vi "_Check range DBL.vi"(6 "Error Mode (Errors)":enum16{"Errors Off", "Errors", "Warnings"}(ring)=enum."Errors", 7 "Range Table Identifier":string, 8 "error in (no error)":errorcluster, 10 "DBL Value In":dbl, 11 "VISA resource name":refnum<visa-resource-name>) -> (0 "error out":errorcluster, 2 "DBL Value Out":dbl, 3 "VISA resource name out":refnum<visa-resource-name>)   [LabVIEW 2015, in "Rohde&Schwarz CMXP NR FR2 Measurement.lvlib"]
uses:
  <instrlib>/Rohde&Schwarz CMXP NR FR2 Measurement/Rohde&Schwarz CMXP NR FR2 Measurement.lvlib
  <instrlib>/Rohde&Schwarz CMXP NR FR2 Measurement/Private/rsidr_core.llb/type_Error_Codes.ctl
  <instrlib>/Rohde&Schwarz CMXP NR FR2 Measurement/Public/Utility/rsidr_core_global.vi
  <instrlib>/Rohde&Schwarz CMXP NR FR2 Measurement/Private/rsidr_core.llb/rsidr_core.lvlib
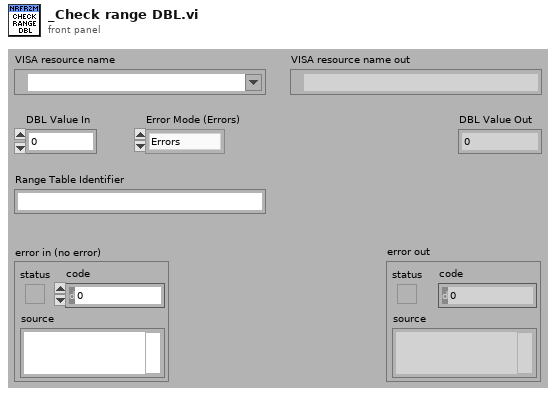
[diagram p1: front panel]
types:
  T1 = typedef "Rohde&Schwarz CMXP NR FR2 Measurement.lvlib/rsidr_core.lvlib/type_Error_Codes.ctl" = enum16{"No_error", "VISA_err_ResourceNotFound", "VISA_err_Timeout", "VISA_warn_MoreDataAvailable", "RS_err_MissingCallback", "RS_err_InvalidAttribute", "RS_err_InvalidValue", "RS_err_UnknownResource", "RS_err_AlreadyInitialized", "RS_err_InstrumentStatus", "RS_err_BadRepCapName", "RS_err_TypesMismatch", "RS_err_ValueNotSupported", "RS_err_InvalidRngTable", "RS_err_IDqueryFail", "RS_err_UnexpResponse", "VISA_warn_ConfigNotLoaded", "RS_err_AttributeNotReadable", "RS_err_AttributeNotWritable", "RS_err_InstrumentType", "RS_err_InstrumentOption", "VISA_err_InvalidSize", "RS_err_ReliabilityIndicator", "VISA_warn_UnknownStatus", "VISA_warn_TermCharRead", "VISA_err_IO_error", "RS_err_FunctionNotSupported", "VISA_warn_QueueEmpty"}
  T2 = cluster{"Name":string, "Type":enum16{"Range", "Coerced", "Discrete"}, "Entries":cluster{"Name":string, "Discrete or Min":dbl, "Max":dbl, "Coerced":dbl, "Command":string}[]}[]
  T3 = cluster{"Name":string, "Discrete or Min":dbl, "Max":dbl, "Coerced":dbl, "Command":string}[]
  T4 = cluster{"Name":string, "Discrete or Min":dbl, "Max":dbl, "Coerced":dbl, "Command":string}
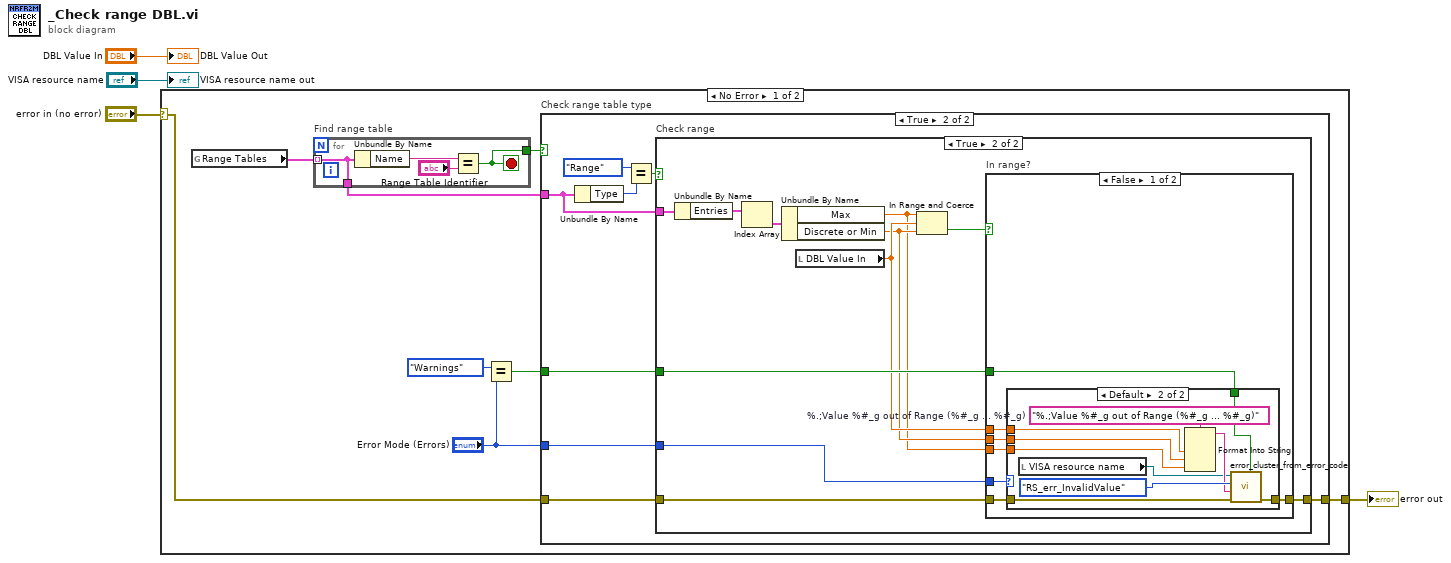
[diagram p0: block diagram]
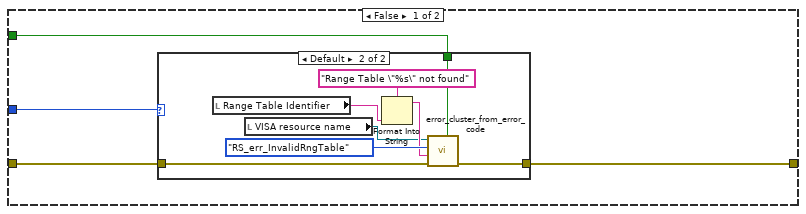
[diagram p2: hidden frame]
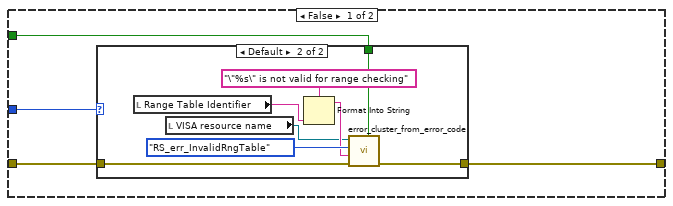
[diagram p4: hidden frame]
diagram:
  n1 = case shown="No Error" "error in (no error)" {
    selector: "error in (no error)" -> [w9 w81]
    tunnel: [w8 w81] -> w2
    frame No Error {
      n2 = global read "rsidr_core_global.vi" "Range Tables"() -> (w12:T2)
      n3 = for "Find range table" {
        tunnel: w12 -> [w78] mode=indexing
        tunnel: [w78] -> w11
        tunnel: [w77] -> w10
        stop <- w77 stop-if-true
        n4 = Unbundle By Name(w78) -> ("Name"=w79:string)
        n5 = Equal?(x=w79, y="Range Table Identifier") -> (x = y?=w77:bool)
      }
      n6 = Equal?(x=enum16{"Errors Off", "Errors", "Warnings"}."Warnings" ("Error Mode"), y="Error Mode (Errors)") -> (x = y?=w5:bool)
      n7 = case "Check range table type" shown="True" w10 {
        tunnel: w11 -> [_ w28]
        tunnel: w9 -> [w16 w31]
        tunnel: [w15 w30] -> w8
        tunnel: "Error Mode (Errors)" -> [w14 w27]
        tunnel: w5 -> [w13 w26]
        frame False {
          n8 = case shown="Default" w14 {
            tunnel: w16 -> [w17 w21]
            tunnel: [w17 w20] -> w15
            tunnel: w13 -> [_ w19]
            frame "Errors Off" {
            }
            frame Default {
              n9 = local read "Range Table Identifier"() -> (w25:string)
              n10 = local read "VISA resource name"() -> (w18:refnum<visa-resource-name>)
              n11 = Format Into String(format string="Range Table \"%s\" not found", w25) -> (resulting string=w22:string)  [unwired: 2 in, 1 out]
              n12 = call <instrlib>:"error_cluster_from_error_code.vi"("is warning? (False)"=w19, "error in"=w21, "error message (\"\")"=w22, "Error Enum in"=type_Error_Codes."RS_err_InvalidRngTable", "VISA resource name"=w18) -> ("error out"=w20:errorcluster)  [unwired: 5 in, 1 out]
            }
          }
        }
        frame True {
          n13 = Unbundle By Name(w28) -> ("Type"=w33:enum16{"Range", "Coerced", "Discrete"})
          n14 = Equal?(x=enum16{"Range", "Coerced", "Discrete"}."Range" ("Type"), y=w33) -> (x = y?=w29:bool)
          n15 = case "Check range" shown="True" w29 {
            tunnel: w31 -> [w37 w56]
            tunnel: [w36 w55] -> w30
            tunnel: w28 -> [_ w57]
            tunnel: w27 -> [w35 w54]
            tunnel: w26 -> [w34 w53]
            frame False {
              n16 = case shown="Default" w35 {
                tunnel: w37 -> [w38 w42]
                tunnel: [w38 w41] -> w36
                tunnel: w34 -> [_ w40]
                frame "Errors Off" {
                }
                frame Default {
                  n17 = local read "Range Table Identifier"() -> (w46:string)
                  n18 = local read "VISA resource name"() -> (w39:refnum<visa-resource-name>)
                  n19 = Format Into String(format string="\"%s\" is not valid for range checking", w46) -> (resulting string=w43:string)  [unwired: 2 in, 1 out]
                  n20 = call <instrlib>:"error_cluster_from_error_code.vi"("is warning? (False)"=w40, "error in"=w42, "error message (\"\")"=w43, "Error Enum in"=type_Error_Codes."RS_err_InvalidRngTable", "VISA resource name"=w39) -> ("error out"=w41:errorcluster)  [unwired: 5 in, 1 out]
                }
              }
            }
            frame True {
              n21 = Unbundle By Name(w57) -> ("Entries"=w52:T3)
              n22 = Index Array(array=w52) -> (element=w51:T4)  [unwired: 1 in]
              n23 = Unbundle By Name(w51) -> ("Max"=w47:dbl, "Discrete or Min"=w48:dbl)
              n24 = local read "DBL Value In"() -> (w49:dbl)
              n25 = In Range and Coerce(upper limit=w47, x=w49, lower limit=w48) -> (In Range?=w50:bool)  [unwired: 1 out]
              n26 = case "In range?" shown="False" w50 {
                tunnel: w56 -> [w64 w76]
                tunnel: [w63 w76] -> w55
                tunnel: w54 -> [w62 _]
                tunnel: w53 -> [w61 _]
                tunnel: w49 -> [w60 _]
                tunnel: w48 -> [w59 _]
                tunnel: w47 -> [w58 _]
                frame False {
                  n27 = case shown="Default" w62 {
                    tunnel: w64 -> [w65 w73]
                    tunnel: [w65 w72] -> w63
                    tunnel: w61 -> [_ w71]
                    tunnel: w60 -> [_ w68]
                    tunnel: w59 -> [_ w67]
                    tunnel: w58 -> [_ w66]
                    frame "Errors Off" {
                    }
                    frame Default {
                      w69 = "%.;Value %#_g out of Range (%#_g ... %#_g)"  # %.;Value %#_g out of Range (%#_g ... %#_g)
                      n28 = local read "VISA resource name"() -> (w70:refnum<visa-resource-name>)
                      n29 = Format Into String(format string=w69, w68, w67, w66) -> (resulting string=w74:string)  [unwired: 2 in, 1 out]
                      n30 = call <instrlib>:"error_cluster_from_error_code.vi"("is warning? (False)"=w71, "error in"=w73, "error message (\"\")"=w74, "Error Enum in"=type_Error_Codes."RS_err_InvalidValue", "VISA resource name"=w70) -> ("error out"=w72:errorcluster)  [unwired: 5 in, 1 out]
                    }
                  }
                }
                frame True {
                }
              }
            }
          }
        }
      }
    }
    frame Error {
    }
  }
  "error out" <- w2
  "VISA resource name out" <- "VISA resource name"
  "DBL Value Out" <- "DBL Value In"
